vi "logic_mux.vi"(1 "C":T1, 2 "R-1":T2, 3 "B":bool, 4 "A":bool) -> (0 "R":bool)   [LabVIEW 2013]
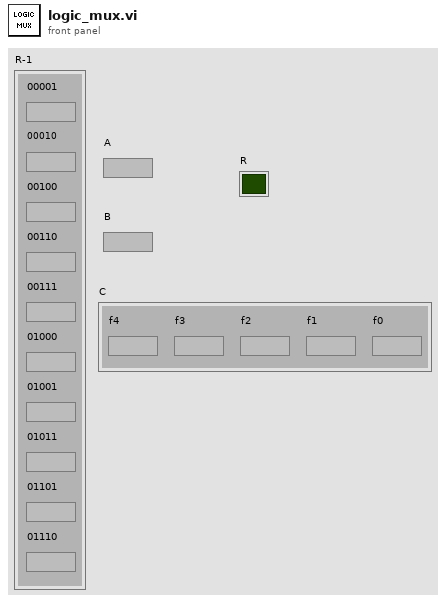
[diagram p1: front panel]
types:
  T1 = cluster{"f4":bool, "f3":bool, "f2":bool, "f1":bool, "f0":bool}
  T2 = cluster{"00001":bool, "00010":bool, "00100":bool, "00110":bool, "00111":bool, "01000":bool, "01001":bool, "01011":bool, "01101":bool, "01110":bool}
  T3 = cluster{"01000":bool, "01001":bool, "01011":bool, "01101":bool, "01110":bool}
  T4 = cluster{bool, bool, bool, bool, bool, bool, bool, bool}
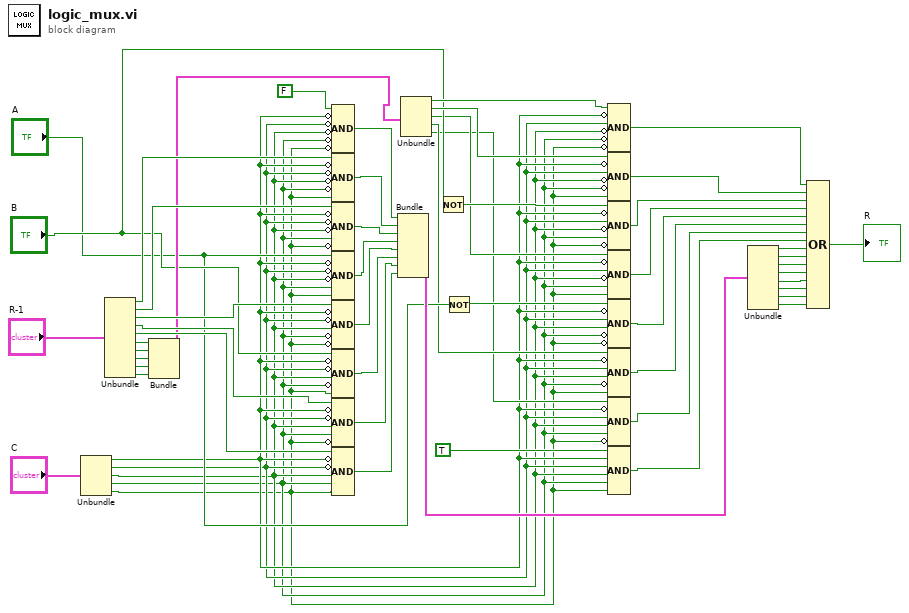
[diagram p0: block diagram]
diagram:
  n1 = Unbundle("C") -> ("f4"=w5:bool, "f3"=w4:bool, "f2"=w3:bool, "f1"=w2:bool, "f0"=w1:bool)
  n2 = Unbundle("R-1") -> ("00001"=w26:bool, "00010"=w25:bool, "00100"=w24:bool, "00110"=w23:bool, "00111"=w22:bool, "01000"=w17:bool, "01001"=w18:bool, "01011"=w19:bool, "01101"=w20:bool, "01110"=w21:bool)
  n3 = Bundle("01000"=w17, "01001"=w18, "01011"=w19, "01101"=w20, "01110"=w21) -> (w16:T3)  [unwired: 1 in]
  n4 = Compound Arithmetic op=AND(FALSE, invert w5, invert w4, invert w3, invert w2, invert w1) -> (w52:bool)
  n5 = Compound Arithmetic op=AND(w26, invert w5, invert w4, invert w3, invert w2, w1) -> (w51:bool)
  n6 = Compound Arithmetic op=AND(w25, invert w5, invert w4, invert w3, w2, invert w1) -> (w50:bool)
  n7 = Compound Arithmetic op=AND("A", invert w5, invert w4, invert w3, w2, w1) -> (w49:bool)
  n8 = Compound Arithmetic op=AND(w24, invert w5, invert w4, w3, invert w2, invert w1) -> (w48:bool)
  n9 = Compound Arithmetic op=AND("B", invert w5, invert w4, w3, invert w2, w1) -> (w47:bool)
  n10 = Compound Arithmetic op=AND(w23, invert w5, invert w4, w3, w2, invert w1) -> (w46:bool)
  n11 = Compound Arithmetic op=AND(w22, invert w5, invert w4, w3, w2, w1) -> (w45:bool)
  n12 = Bundle(w52, w51, w50, w49, w48, w47, w46, w45) -> (w36:T4)  [unwired: 1 in]
  n13 = Unbundle(w16) -> ("01000"=w15:bool, "01001"=w14:bool, "01011"=w11:bool, "01101"=w8:bool, "01110"=w7:bool)
  n14 = Not(x="B") -> (.not. x?=w13:bool)
  n15 = Not(x="A") -> (.not. x?=w10:bool)
  n16 = Compound Arithmetic op=AND(w15, invert w5, w4, invert w3, invert w2, invert w1) -> (w44:bool)
  n17 = Compound Arithmetic op=AND(w14, invert w5, w4, invert w3, invert w2, w1) -> (w43:bool)
  n18 = Compound Arithmetic op=AND(w13, invert w5, w4, invert w3, w2, invert w1) -> (w42:bool)
  n19 = Compound Arithmetic op=AND(w11, invert w5, w4, invert w3, w2, w1) -> (w41:bool)
  n20 = Compound Arithmetic op=AND(w10, invert w5, w4, w3, invert w2, invert w1) -> (w40:bool)
  n21 = Compound Arithmetic op=AND(w8, invert w5, w4, w3, invert w2, w1) -> (w39:bool)
  n22 = Compound Arithmetic op=AND(w7, invert w5, w4, w3, w2, invert w1) -> (w38:bool)
  n23 = Compound Arithmetic op=AND(TRUE, w5, w4, w3, w2, w1) -> (w37:bool)
  n24 = Unbundle(w36) -> (w35:bool, w34:bool, w33:bool, w32:bool, w31:bool, w30:bool, w29:bool, w28:bool)
  n25 = Compound Arithmetic op=OR(w44, w43, w42, w41, w40, w39, w38, w37, w35, w34, w33, w32, w31, w30, w29, w28) -> (→"R":bool)
